vi "PartInfo_Algo.vi"(8 "error in (no error)":errorcluster, 10 "PartDetails":T1, 11 "Algorithm in":refnum<class "Algorithm.lvclass">) -> (0 "error out":errorcluster, 3 "Algorithm out":refnum<class "Algorithm.lvclass">)   [LabVIEW 2019, in "Algorithm.lvclass"]
uses:
  FrameworkOverrides/Algorithm.lvclass
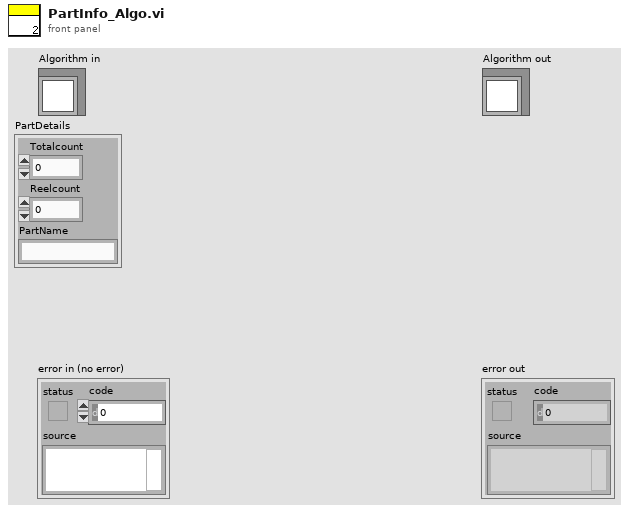
[diagram p1: front panel]
types:
  T1 = cluster{"Totalcount":u64, "Reelcount":u64, "PartName":string}
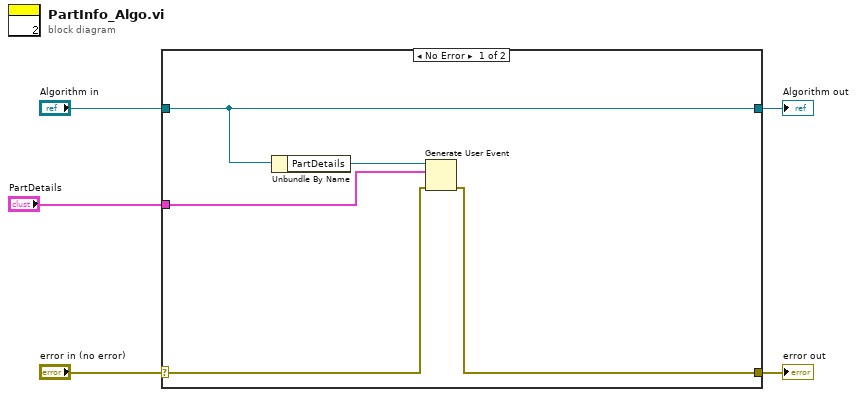
[diagram p0: block diagram]
diagram:
  n1 = case shown="No Error" "error in (no error)" {
    selector: "error in (no error)" -> [w8 w12]
    tunnel: [w7 w12] -> w4
    tunnel: [w10 w11] -> w2
    tunnel: "Algorithm in" -> [w10 w11]
    tunnel: "PartDetails" -> [w6 _]
    frame No Error {
      n2 = Unbundle By Name(w10) -> ("PartDetails"=w9:refnum<user-event>)
      n3 = Generate User Event(user event=w9, event data cluster=w6, error in=w8) -> (error out=w7:errorcluster)  [unwired: 1 in, 1 out]
    }
    frame Error {
    }
  }
  "error out" <- w4
  "Algorithm out" <- w2
